vi "thermal simulator kernel.vi"(0 "Power":dbl=0.3259911894273128 format="%#_4g", 1 "tau":i32=80, 2 "P delay center":enum16{"1", "2", "3", "4", "5", "6", "7"}(ring)=enum."4" caption="del", 5 "K":dbl=65.0, 7 "T air":dbl=20.0, 9 "B":dbl=0.05, 11 "air speed":dbl, 12 "A":dbl=0.01, 13 "insulation":enum16{"uncovered", "covered"}(ring)=enum."covered") -> (4 "P eff":dbl=0.32599118942731276 format="%#_4g", 8 "Temp":dbl=41.19014686638811 format="%#_4g")   [LabVIEW 2016]
doc: "this vi simulates the thermal response of the bug during a given time step\n\nPaul K Dixon\nCSUSB Physics"
uses:
  <vilib>/ptbypt/NI_PtbyPt.lvlib
panel:
  out "delta T":dbl=21.190146866388112 format="%#.3f"
  # "Bug Thermal Simulator"
  # "tuning parameters"
  # "environmental factors"
  # "intermediate responses"
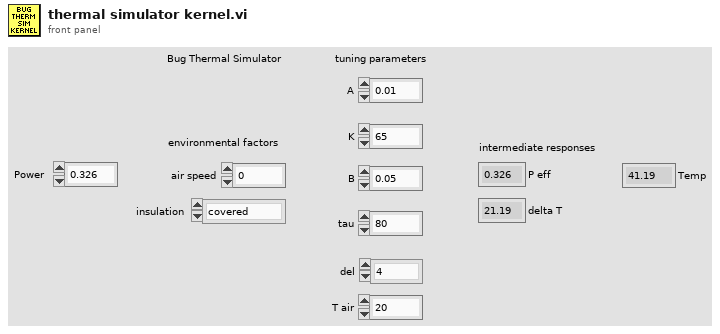
[diagram p1: front panel]
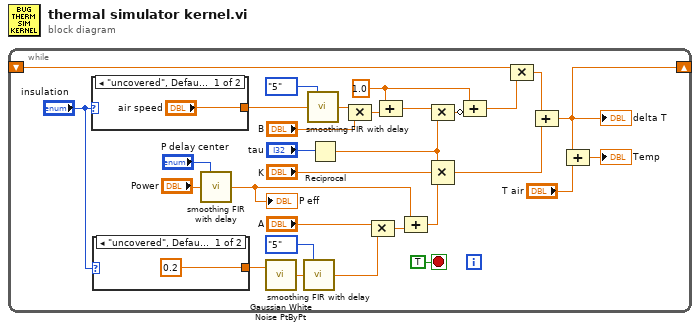
[diagram p0: block diagram]
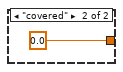
[diagram p2: hidden frame]
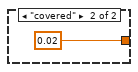
[diagram p3: hidden frame]
diagram:
  n1 = while {
    shift-right: [w12] -> _
    shift-left: _ -> [w17]
    stop <- TRUE stop-if-true
    w18 = 1.0
    n2 = case shown="\"uncovered\", Default" "insulation" {
      tunnel: ["air speed" 0.0 ("standard deviation")] -> w2
      frame "uncovered", Default {
      }
      frame "covered" {
      }
    }
    n3 = case shown="\"uncovered\", Default" "insulation" {
      tunnel: [0.2 ("standard deviation") 0.02 ("standard deviation")] -> w3
      frame "uncovered", Default {
      }
      frame "covered" {
      }
    }
    n4 = call "smoothing FIR with delay.vi"("delay"="P delay center", "x in"="Power") -> ("x out"=w4:dbl)  [unwired: 13 in]
    "P eff" <- w4
    n5 = call <vilib>:"Gaussian White Noise PtByPt.vi"("standard deviation"=w3) -> ("Gaussian white noise"=w8:dbl)  [unwired: 2 in]
    n6 = call "smoothing FIR with delay.vi"("delay"=enum16{"1", "2", "3", "4", "5", "6", "7"}."5" ("delay center"), "x in"=w8) -> ("x out"=w7:dbl)  [unwired: 13 in]
    n7 = call "smoothing FIR with delay.vi"("delay"=enum16{"1", "2", "3", "4", "5", "6", "7"}."5" ("delay center"), "x in"=w2) -> ("x out"=w11:dbl)  [unwired: 13 in]
    n8 = Reciprocal(x="tau") -> (1/x=w20:dbl)
    n9 = Compound Arithmetic op=MULTIPLY(w11, "B") -> (w29:dbl)
    n10 = Compound Arithmetic op=MULTIPLY("A", w7) -> (w24:dbl)
    n11 = Compound Arithmetic op=ADD(w18, w29) -> (w21:dbl)
    n12 = Compound Arithmetic op=ADD(w4, w24) -> (w22:dbl)
    n13 = Compound Arithmetic op=MULTIPLY(w21, w20) -> (w19:dbl)
    n14 = Compound Arithmetic op=MULTIPLY(w20, "K", w22) -> (w16:dbl)
    n15 = Compound Arithmetic op=ADD(w18, invert w19) -> (w14:dbl)
    n16 = Compound Arithmetic op=MULTIPLY(w17, w14) -> (w13:dbl)
    n17 = Compound Arithmetic op=ADD(w13, w16) -> (w12:dbl)
    "delta T" <- w12
    n18 = Compound Arithmetic op=ADD(w12, "T air") -> (→"Temp":dbl)
  }
